vi "Autonomous Independent.vi"   [LabVIEW 2015]
doc: "This VI is called when autonomous begins, and will automatically be terminated when autonomous ends. You can carry out timed or sensor driven robot movement independently without needing to return to the caller."
uses:
  <vilib>/Rock Robotics/WPI/Solenoid/WPI_SolenoidValue.ctl
  <vilib>/Rock Robotics/WPI/Utilities/WPI_GetSetVariantRefNum.vi
  <vilib>/Rock Robotics/Network Tables/NT Read String.vi
  <vilib>/Rock Robotics/WPI/Solenoid/WPI_SolenoidSetEnum.vi
panel:
  # "Be sure to right-click and choose Data Operations>>Make Current Value default if you want to save the array values with the VI"
types:
  T1 = typedef "WPI_RobotDriveDevRef.ctl" = cluster{"DevStatus":errorcluster, "Motors[]":T2[], "Square Inputs":bool, "Max Output":dbl}
  T2 = typedef "WPI_MotorControlDeviceRef.ctl" = cluster{"DeviceStatus":errorcluster, "Type":T3, "PWM":cluster{"PWM Channel":T4, "DeadBand":T5}, "CAN":cluster{"Device Number":u8, "Control Mode":T6, "Semaphore":T7, "Max Vout":dbl, "TalonSRX Control Mode":T8}, "Invert":bool}
  T3 = typedef "WPI_MotorControlType.ctl" = enum16{"PWM", "CAN", "CANTalonSRX"}
  T4 = typedef "FPGA_DIOPWMChannel.ctl" = enum8{"PWM 0", "PWM 1", "PWM 2", "PWM 3", "PWM 4", "PWM 5", "PWM 6", "PWM 7", "PWM 8", "PWM 9", "PWM MXP 0", "PWM MXP 1", "PWM MXP 2", "PWM MXP 3", "PWM MXP 4", "PWM MXP 5", "PWM MXP 6", "PWM MXP 7", "PWM MXP 8", "PWM MXP 9", "Invalid"}
  T5 = typedef "WPI_PWMDeadband.ctl" = cluster{"Name":string, "maxPositivePwm":i32, "minPositivePwm":i32, "centerPwm":i32, "maxNegativePwm":i32, "minNegativePwm":i32, "angularRange":u16}
  T6 = typedef "WPI_CANJaguar_ControlMode.ctl" = enum8{"Percent VBus", "Current", "Speed", "Position", "Voltage"}
  T7 = typedef "Semaphore RefNum" = refnum<k1>
  T8 = typedef "WPI_CANTalonSRX_APIControlMode.ctl" = enum8{"Percent VBus", "Speed", "Position", "Slave", "Unchanged / Invalid", "Voltage Compensation", "Current", "Motion Profile"}
  T9 = typedef "WPI_SolenoidValue.ctl" = enum16{"Off", "On", "Forward", "Reverse"}
  T10 = typedef "WPI_SolenoidDevRef.ctl" = cluster{"DevStatus":errorcluster, "Pneumatics Control Module":u8, "Forward Solenoid Channel":T11, "Reverse Solenoid Channel":T11}
  T11 = typedef "WPI_SolenoidChannel.ctl" = enum8{"Solenoid 0", "Solenoid 1", "Solenoid 2", "Solenoid 3", "Solenoid 4", "Solenoid 5", "Solenoid 6", "Solenoid 7", "Invalid"}
  T12 = typedef "WPI_AccelerometerDevRef.ctl" = cluster{"DevStatus":errorcluster, "Scaling":T13, "Analog Channels":T14, "I2C Bus":T16, "SPI Bus":T17, "Accel Range":T18, "ADXL Axes":T19, "Handle":i32, "Device Address":u8, "Accel Type":enum16{"Analog", "ADXL345 I2C", "ADXL345 SPI", "Internal", "ADXL362 SPI"}}
  T13 = typedef "WPI_AccelerometerScaling.ctl" = cluster{"Gain (VoltsPerG)":dbl, "Center Voltage":dbl}
  T14 = typedef "WPI_AccelerometerAnalogChannels.ctl" = cluster{"X-Axis":T15, "Y-Axis":T15, "Z-Axis":T15}
  T15 = typedef "FPGA_AIChannel.ctl" = enum8{"AI 0", "AI 1", "AI 2", "AI 3", "AI MXP 0", "AI MXP 1", "AI MXP 2", "AI MXP 3", "Invalid"}
  T16 = typedef "i2c_bus.ctl" = enum16{"I2C On-Board", "I2C MXP", "Invalid"}
  T17 = typedef "spi_bus.ctl" = enum16{"SPI On-Board, CS0", "SPI On-Board, CS1", "SPI On-Board, CS2", "SPI On-Board, CS3", "SPI MXP", "Invalid"}
  T18 = typedef "ADXL345 Range.ctl" = u8
  T19 = typedef "WPI_AccelerometerADXL345 Axes.ctl" = cluster{"X-Axis":bool, "Y-Axis":bool, "Z-Axis":bool}
  T20 = cluster{"X-Axis":dbl, "Y-Axis":dbl, "Z-Axis":dbl}
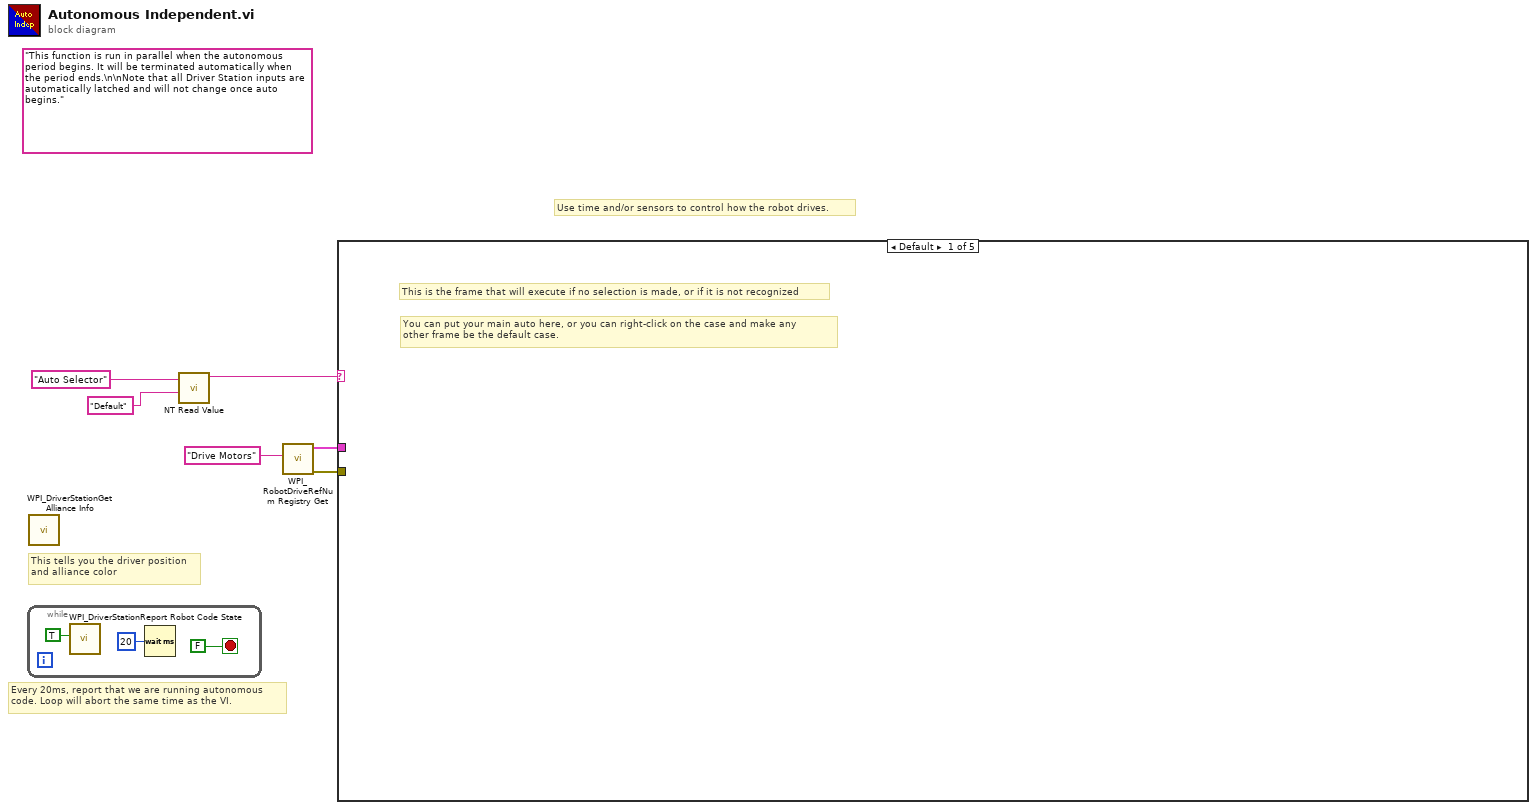
[diagram p0: block diagram]
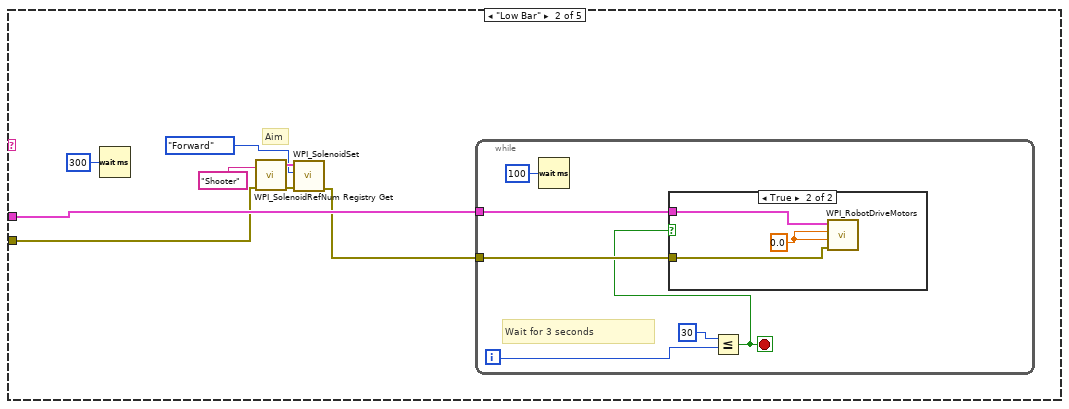
[diagram p2: hidden frame]
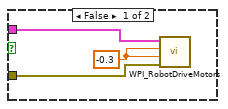
[diagram p3: hidden frame]
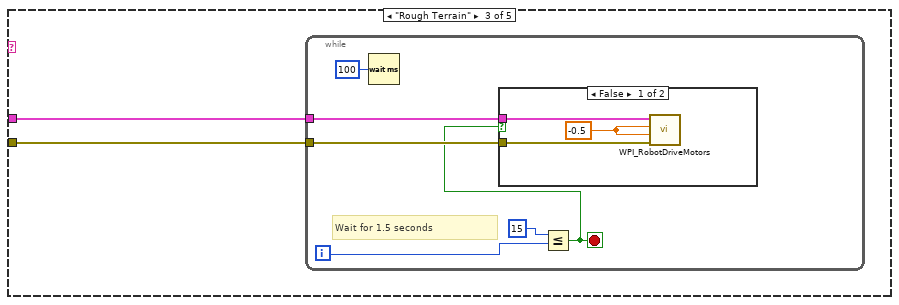
[diagram p4: hidden frame]
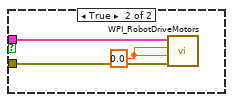
[diagram p5: hidden frame]
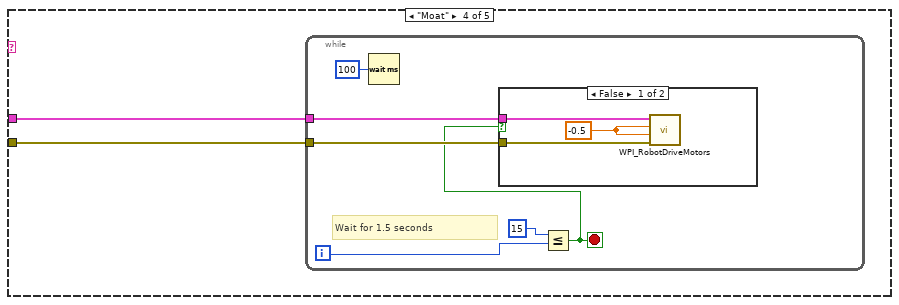
[diagram p6: hidden frame]
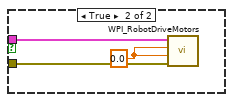
[diagram p7: hidden frame]
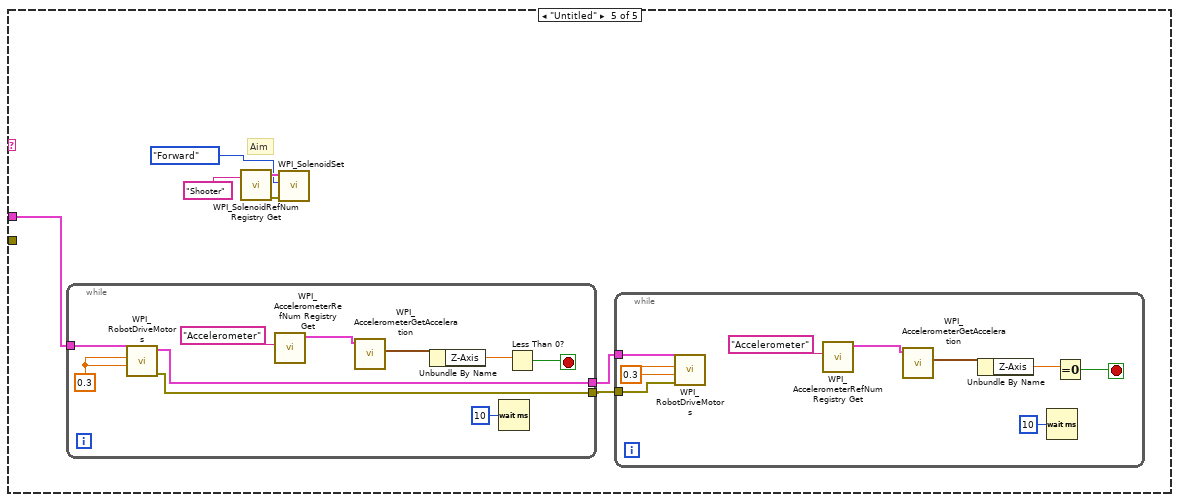
[diagram p8: hidden frame]
diagram:
  (unwired) "This function is run in parallel when the autonomous period begins. It will be terminated automatically when the period ends.\n\nNote that all Driver Station inputs are automatically latched and will not change once auto begins."
  # "Every 20ms, report that we are running autonomous\ncode. Loop will abort the same time as the VI."
  # "Use time and/or sensors to control how the robot drives."
  # "This tells you the driver position\nand alliance color"
  n1 = while {
    stop <- FALSE stop-if-true
    n2 = call <vilib>:"WPI_DriverStationReport Robot Code State.vi"("Autonomous"=TRUE) -> ()  [unwired: 10 in, 1 out]
    n3 = Wait (ms)(milliseconds to wait=u32 20) -> ()  [unwired: 1 out]
  }
  n4 = call <vilib>:"WPI_DriverStationGet Alliance Info.vi"() -> ()  [unwired: 12 out]
  n5 = call-poly <vilib>:"NT Read Value.vi"("Default Value"="Default", "Name"="Auto Selector") -> ("String"=w5:string)  [unwired: 8 in, 1 out]
  n6 = call <vilib>:"WPI_RobotDriveRefNum Registry Get.vi"("refnum name"="Drive Motors") -> ("error out"=w1:errorcluster, "RobotDriveDevRef"=w4:T1)  [unwired: 9 in]
  n7 = case shown="Default" w5 {
    tunnel: w4 -> [_ w17 w31 w45 w62]
    tunnel: w1 -> [_ w11 w30 w44 _]
    frame Default {
      # "You can put your main auto here, or you can right-click on the case and make any\nother frame be the default case."
      # "This is the frame that will execute if no selection is made, or if it is not recognized"
    }
    frame "Low Bar" {
      # "Aim"
      n8 = Wait (ms)(milliseconds to wait=u32 300) -> ()  [unwired: 1 out]
      n9 = call <vilib>:"WPI_SolenoidRefNum Registry Get.vi"("error in (no error)"=w11, "refnum name"="Shooter") -> ("error out"=w15:errorcluster, "SolenoidDevRef"=w16:T10)  [unwired: 8 in]
      n10 = call-poly <vilib>:"WPI_SolenoidSet.vi"("error in (no error)"=w15, "Value"=WPI_SolenoidValue."Forward", "SolenoidDevRef"=w16) -> ("error out"=w10:errorcluster)  [unwired: 7 in, 1 out]
      n11 = while {
        tunnel: w17 -> [w20]
        tunnel: w10 -> [w19]
        i -> [w22]
        stop <- w18 stop-if-true
        # "Wait for 3 seconds"
        n12 = Wait (ms)(milliseconds to wait=u32 100) -> ()  [unwired: 1 out]
        n13 = Less Or Equal?(x=w22, y=30) -> (x <= y?=w18:bool)
        n14 = case shown="True" w18 {
          tunnel: w20 -> [w25 w28]
          tunnel: w19 -> [w24 w27]
          frame False {
            w26 = -0.3 ("LeftSpeed")
            n15 = call <vilib>:"WPI_RobotDriveMotors.vi"("error in (no error)"=w24, "RightSpeed"=w26, "LeftSpeed"=w26, "RobotDriveDevRef"=w25) -> ()  [unwired: 5 in, 3 out]
          }
          frame True {
            w29 = 0.0 ("LeftSpeed")
            n16 = call <vilib>:"WPI_RobotDriveMotors.vi"("error in (no error)"=w27, "RightSpeed"=w29, "LeftSpeed"=w29, "RobotDriveDevRef"=w28) -> ()  [unwired: 5 in, 3 out]
          }
        }
      }
    }
    frame "Rough Terrain" {
      n17 = while {
        tunnel: w31 -> [w34]
        tunnel: w30 -> [w33]
        i -> [w36]
        stop <- w32 stop-if-true
        # "Wait for 1.5 seconds"
        n18 = Wait (ms)(milliseconds to wait=u32 100) -> ()  [unwired: 1 out]
        n19 = Less Or Equal?(x=w36, y=15) -> (x <= y?=w32:bool)
        n20 = case shown="False" w32 {
          tunnel: w34 -> [w39 w42]
          tunnel: w33 -> [w38 w41]
          frame False {
            w40 = -0.5 ("LeftSpeed")
            n21 = call <vilib>:"WPI_RobotDriveMotors.vi"("error in (no error)"=w38, "RightSpeed"=w40, "LeftSpeed"=w40, "RobotDriveDevRef"=w39) -> ()  [unwired: 5 in, 3 out]
          }
          frame True {
            w43 = 0.0 ("LeftSpeed")
            n22 = call <vilib>:"WPI_RobotDriveMotors.vi"("error in (no error)"=w41, "RightSpeed"=w43, "LeftSpeed"=w43, "RobotDriveDevRef"=w42) -> ()  [unwired: 5 in, 3 out]
          }
        }
      }
    }
    frame "Moat" {
      n23 = while {
        tunnel: w45 -> [w48]
        tunnel: w44 -> [w47]
        i -> [w50]
        stop <- w46 stop-if-true
        # "Wait for 1.5 seconds"
        n24 = Wait (ms)(milliseconds to wait=u32 100) -> ()  [unwired: 1 out]
        n25 = Less Or Equal?(x=w50, y=15) -> (x <= y?=w46:bool)
        n26 = case shown="False" w46 {
          tunnel: w48 -> [w53 w56]
          tunnel: w47 -> [w52 w55]
          frame False {
            w54 = -0.5 ("LeftSpeed")
            n27 = call <vilib>:"WPI_RobotDriveMotors.vi"("error in (no error)"=w52, "RightSpeed"=w54, "LeftSpeed"=w54, "RobotDriveDevRef"=w53) -> ()  [unwired: 5 in, 3 out]
          }
          frame True {
            w57 = 0.0 ("LeftSpeed")
            n28 = call <vilib>:"WPI_RobotDriveMotors.vi"("error in (no error)"=w55, "RightSpeed"=w57, "LeftSpeed"=w57, "RobotDriveDevRef"=w56) -> ()  [unwired: 5 in, 3 out]
          }
        }
      }
    }
    frame "Untitled" {
      # "Aim"
      n29 = while {
        tunnel: w62 -> [w83]
        tunnel: [w75] -> w64
        tunnel: [w74] -> w63
        stop <- w77 stop-if-true
        w82 = 0.3 ("LeftSpeed")
        n30 = call <vilib>:"WPI_RobotDriveMotors.vi"("RightSpeed"=w82, "LeftSpeed"=w82, "RobotDriveDevRef"=w83) -> ("error out"=w74:errorcluster, "RobotDriveDevRef"=w75:T1)  [unwired: 6 in, 1 out]
        n31 = call <vilib>:"WPI_AccelerometerRefNum Registry Get.vi"("refnum name"="Accelerometer") -> ("AccelerometerDevRef"=w80:T12)  [unwired: 9 in, 1 out]
        n32 = call <vilib>:"WPI_AccelerometerGetAcceleration.vi"("AccelerometerDevRef"=w80) -> ("Accelerations"=w79:T20)  [unwired: 8 in, 2 out]
        n33 = Unbundle By Name(w79) -> ("Z-Axis"=w78:dbl)
        n34 = Wait (ms)(milliseconds to wait=u32 10) -> ()  [unwired: 1 out]
        n35 = Less Than 0?(x=w78) -> (x < 0?=w77:bool)
      }
      n36 = call <vilib>:"WPI_SolenoidRefNum Registry Get.vi"("refnum name"="Shooter") -> ("error out"=w60:errorcluster, "SolenoidDevRef"=w61:T10)  [unwired: 9 in]
      n37 = call-poly <vilib>:"WPI_SolenoidSet.vi"("error in (no error)"=w60, "Value"=WPI_SolenoidValue."Forward", "SolenoidDevRef"=w61) -> ()  [unwired: 7 in, 2 out]
      n38 = while {
        tunnel: w64 -> [w73]
        tunnel: w63 -> [w65]
        stop <- w67 stop-if-true
        w72 = 0.3 ("LeftSpeed")
        n39 = call <vilib>:"WPI_RobotDriveMotors.vi"("error in (no error)"=w65, "RightSpeed"=w72, "LeftSpeed"=w72, "RobotDriveDevRef"=w73) -> ()  [unwired: 5 in, 3 out]
        n40 = call <vilib>:"WPI_AccelerometerRefNum Registry Get.vi"("refnum name"="Accelerometer") -> ("AccelerometerDevRef"=w70:T12)  [unwired: 9 in, 1 out]
        n41 = call <vilib>:"WPI_AccelerometerGetAcceleration.vi"("AccelerometerDevRef"=w70) -> ("Accelerations"=w69:T20)  [unwired: 8 in, 2 out]
        n42 = Unbundle By Name(w69) -> ("Z-Axis"=w68:dbl)
        n43 = Wait (ms)(milliseconds to wait=u32 10) -> ()  [unwired: 1 out]
        n44 = Equal To 0?(x=w68) -> (x = 0?=w67:bool)
      }
    }
  }
